vi "Log Error.vi"(8 "error in (no error)":errorcluster, 9 "Source":string, 10 "Code":i32, 11 "Error Log Refnum In":refnum<file>) -> (0 "error out":errorcluster, 3 "Error Log Refnum Out":refnum<file>)   [LabVIEW 2020, in "Error Handler.lvlib"]
uses:
  Error Handler.lvlib
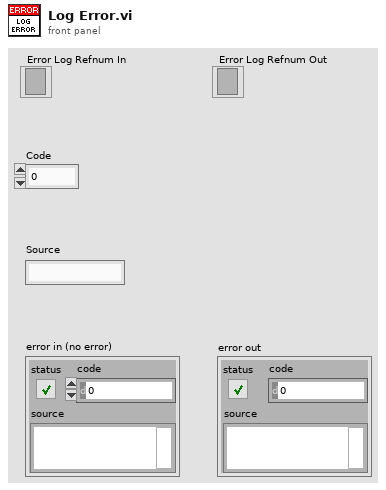
[diagram p1: front panel]
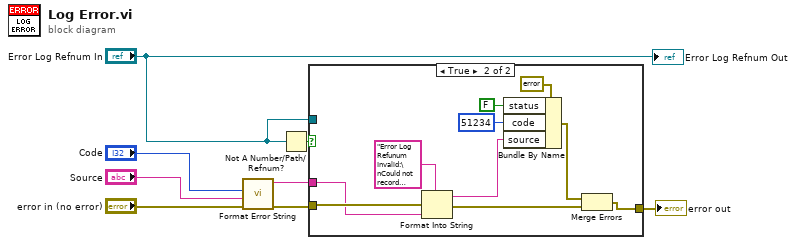
[diagram p0: block diagram]
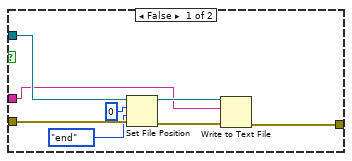
[diagram p2: hidden frame]
diagram:
  n1 = call "Format Error String.vi"("error in (no error)"="error in (no error)", "Source"="Source", "Code"="Code") -> ("error out"=w8:errorcluster, "Error String"=w3:string)  [unwired: 7 in]
  n2 = Not A Number/Path/Refnum?(number/path/refnum="Error Log Refnum In") -> (NaN/Path/Refnum?=w4:bool)
  n3 = case shown="True" w4 {
    tunnel: [w15 w24] -> w2
    tunnel: w8 -> [w14 w26]
    tunnel: "Error Log Refnum In" -> [w13 _]
    tunnel: w3 -> [w9 w17]
    frame False {
      n4 = Set File Position(offset (in bytes) (0)=i64 0, refnum=w13, from (0:start)=enum16{"start", "end", "current"}."end", error in=w14) -> (refnum out=w10:refnum<file>, error out=w16:errorcluster)
      n5 = Write to Text File(file (use dialog)=w10, text=w9, error in=w16) -> (error out=w15:errorcluster)  [unwired: 1 in, 2 out]
    }
    frame True {
      n6 = Format Into String(format string="Error Log Refunum Invalid:\nCould not record error:\n%s", error in=w26, w17) -> (resulting string=w20:string, error out=w23:errorcluster)  [unwired: 1 in]
      n7 = Bundle By Name(cluster=errorcluster {"status"=FALSE, "code"=0, "source"=""} ("error in"), "status"=FALSE, "code"=51234, "source"=w20) -> (w22:errorcluster)
      n8 = Merge Errors(w22, w23) -> (w24:errorcluster)
    }
  }
  "error out" <- w2
  "Error Log Refnum Out" <- "Error Log Refnum In"
